vi "DecorrelationFunction.vi"() -> (1 "waveform":dbl[](array[numeric]), 2 "temporal window (s)":dbl)   [LabVIEW 2013]
uses:
  <vilib>/imath/engines/lvmath2/RunTimeEngine/ErrorHandling/NIMS_Finalize Error.vi
  <vilib>/imath/engines/lvmath2/RunTimeEngine/BuiltInFunctions/nextpowerof2/NIMS_nextpowerof2(GS).vi
  <instcachedir>/0/NIMS_nextpowerof2(GS)_B42BF357393E46BBAF4FDD53A40AE50C.lvgen/NIMS_nextpowerof2(GS)_B42BF357393E46BBAF4FDD53A40AE50C_000.vi
  <vilib>/imath/engines/lvmath2/RunTimeEngine/NodeEndStatement/NIMS_NodeEndStatement_Output.vi
  <instcachedir>/0/NIMS_NodeEndStatement_Output_53EC0D466D134D7ABD903AC30B43404B.lvgen/NIMS_NodeEndStatement_Output_53EC0D466D134D7ABD903AC30B43404B_001.vi
  <instcachedir>/0/NIMS_NodeEndStatement_Output_53EC0D466D134D7ABD903AC30B43404B.lvgen/NIMS_NodeEndStatement_Output_53EC0D466D134D7ABD903AC30B43404B_005.vi
  <vilib>/imath/engines/lvmath2/RunTimeEngine/RangeToken/NIMS_Range.vi
  <instcachedir>/0/NIMS_Range_7481B155BEE341ECA0F59DDB444E2C09.lvgen/NIMS_Range_7481B155BEE341ECA0F59DDB444E2C09_000.vi
  <vilib>/imathl/engines/lvmath/Functions/Error Handling/Create Error.vi
  <vilib>/imath/engines/lvmath2/RunTimeEngine/BuiltInFunctions/length/NIMS_length(GV).vi
  <instcachedir>/0/NIMS_length(GV)_08A3D13377FD4E4B96F5795FBF3698FA.lvgen/NIMS_length(GV)_08A3D13377FD4E4B96F5795FBF3698FA_000.vi
  <vilib>/imath/engines/lvmath2/RunTimeEngine/BuiltInFunctions/rand/NIMS_rand(1,I32).vi
  <vilib>/imath/engines/lvmath2/RunTimeEngine/ErrorHandling/NIMS_Error From Error Code.vi
  <vilib>/imath/engines/lvmath2/RunTimeEngine/ArithmeticOperatorToken/NIMS_ArithmeticOperator_times.vi
  <instcachedir>/0/NIMS_ArithmeticOperator_times_F6527734CE75451889337B8CE94765C6.lvgen/NIMS_ArithmeticOperator_times_F6527734CE75451889337B8CE94765C6_002.vi
  <vilib>/imath/engines/lvmath2/RunTimeEngine/BuiltInFunctions/ifft_shift/NIMS_ifft_shift(GV).vi
  <instcachedir>/0/NIMS_ifft_shift(GV)_21661D804B78421B969BCA642CA10C0F.lvgen/NIMS_ifft_shift(GV)_21661D804B78421B969BCA642CA10C0F_000.vi
  <vilib>/imath/engines/lvmath2/RunTimeEngine/BuiltInFunctions/ifft/NIMS_ifft(CV).vi
  <vilib>/imath/engines/lvmath2/RunTimeEngine/BuiltInFunctions/fftshift/NIMS_fftshift(GV).vi
  <instcachedir>/0/NIMS_fftshift(GV)_BD7A7BA9CA6B470B9A9F73A6A3FEEB3E.lvgen/NIMS_fftshift(GV)_BD7A7BA9CA6B470B9A9F73A6A3FEEB3E_000.vi
  <vilib>/imath/engines/lvmath2/RunTimeEngine/BuiltInFunctions/abs/NIMS_abs(signed).vi
  <instcachedir>/0/NIMS_abs(signed)_C4FCB8E6058B49B797C7C8D53CA5F6EC.lvgen/NIMS_abs(signed)_C4FCB8E6058B49B797C7C8D53CA5F6EC_001.vi
  <vilib>/imath/engines/lvmath2/RunTimeEngine/BuiltInFunctions/max/1 input/NIMS_max(RV).vi
  <instcachedir>/0/NIMS_max(RV)_237633DB1D604D5BA7001287DF3C7957.lvgen/NIMS_max(RV)_237633DB1D604D5BA7001287DF3C7957_000.vi
panel:
  in  "OK Button":bool
  out "noiseBW":dbl
  out "Effective N value (nexpow2)":u32=131072
  out "XY Graph 2":cluster{dbl[], "Windowed X":dbl[]}(graph)
  in  "Fmax":u32=5000
  in  "central frequency (Hz)":dbl=1.0
  out "XY Graph":cluster{dbl[], "Windowed X":dbl[]}(graph)
  in  "Number of data points":u32=131072 min=2 max=131072 step=1
  in  "correlation time (ms)":dbl=1.0
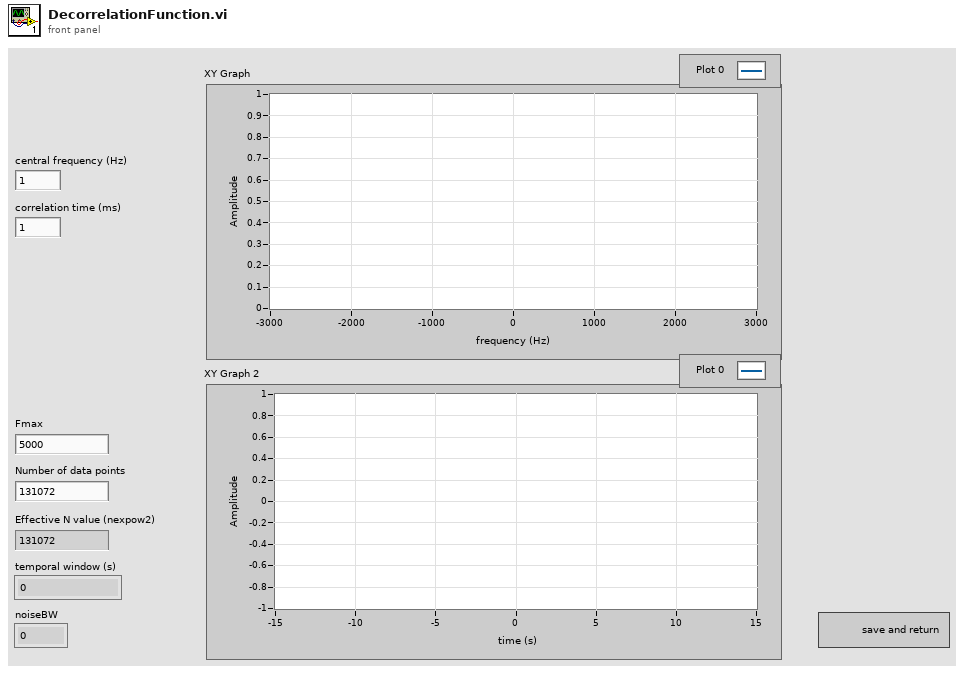
[diagram p1: front panel]
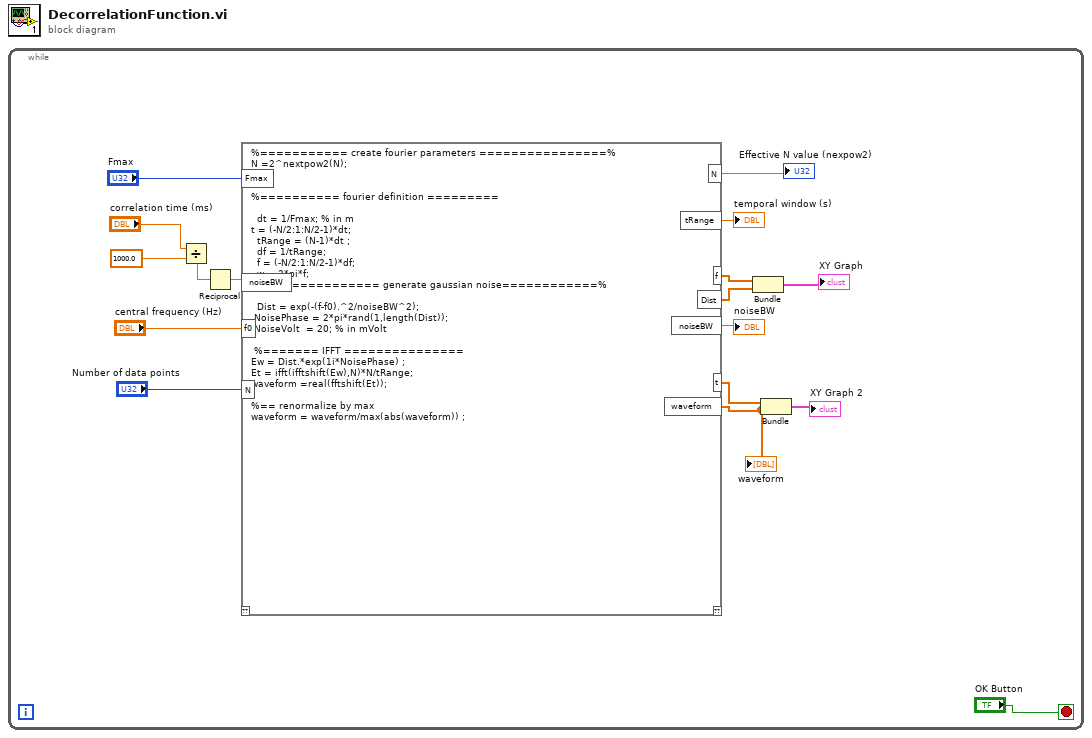
[diagram p0: block diagram]
diagram:
  n1 = while {
    stop <- "OK Button" stop-if-true
    n2 = Divide(x="correlation time (ms)", y=1000.0) -> (x/y=w4:dbl)
    n3 = Reciprocal(x=w4) -> (1/x=w3:dbl)
    n4 = mathscript code="%=========== create fourier parameters ================%\nN =2^nextpow2(N);\n\n\n%========== fourier definition =========\n\n  dt = 1/Fmax; % in m\nt = (-N/2:1:N/2-1)*dt;\n  tRange = (N-1)*dt ;\n  df = 1/tRange;\n  f = (-N/2:1:N/2-1)*df;\n  w = 2*pi*f;\n%=============== generate gaussian noise============%\n \n  Dist = exp(-(f-f0).^2/noiseBW^2);\n NoisePhase = 2*pi*rand(1,length(Dist));\n NoiseVolt  = 20; % in mVolt \n  \n %======= IFFT ===============\nEw = Dist.*exp(1i*NoisePhase) ;\nEt = ifft(ifftshift(Ew),N)*N/tRange;\nwaveform =real(fftshift(Et));\n\n%== renormalize by max\nwaveform = waveform/max(abs(waveform)) ;"("f0"="central frequency (Hz)", "noiseBW"=w3, "N"="Number of data points", "Fmax"="Fmax") -> ("Dist"=w15:dbl[], "f"=w16:dbl[], "t"=w12:dbl[], "waveform"=w11:dbl[], "N"=→"Effective N value (nexpow2)":dbl, "tRange"=→"temporal window (s)":dbl, "noiseBW"=→"noiseBW":dbl)  [unwired: 1 in, 1 out]
    "waveform" <- w11
    n5 = Bundle("f"=w16, "Dist"=w15) -> (→"XY Graph":cluster{"f":dbl[], "Dist":dbl[]})  [unwired: 1 in]
    n6 = Bundle("t"=w12, "waveform"=w11) -> (→"XY Graph 2":cluster{"t":dbl[], "waveform":dbl[]})  [unwired: 1 in]
  }
